vi "TagDB-Load.vi"(8 "error in (no error)":errorcluster, 9 "ignore internal data(T)":bool=TRUE, 10 "file path(empty for default)":path, 11 "DB Ref":refnum<k1>) -> (0 "error out":errorcluster, 1 "version":string, 3 "DB Ref(dup)":refnum<k1>)   [LabVIEW 2017, in "TagDB.lvlib"]
doc: "[Covers: REQ_API_Load]"
uses:
  TagDB.lvlib
  _Support/Disk/tagdbfile-v3.1.ctl
  _Support/Error/_Build Error Cluster.vi
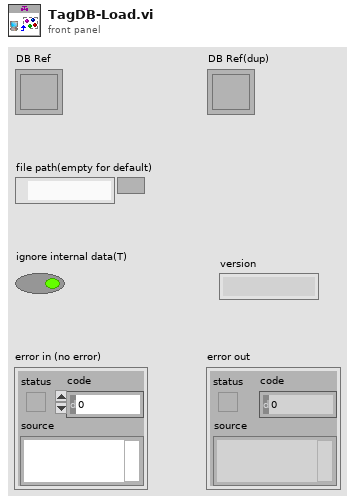
[diagram p1: front panel]
types:
  T1 = typedef "TagDB.lvlib/tagdbfile-v3.1.ctl" = cluster{"version":string, "db":variant[]}
  T2 = enum16{"open", "replace", "create", "open or create", "replace or create", "replace or create with confirmation"}
  T3 = typedef "TagDB.lvlib/tagdb-data.ctl" = cluster{"tag-map":variant, "timestamp-map":variant, "namecacher-map":variant, "DataTypeCacher-map":variant, "Tag Adding Lock?":bool, "Global Change Timestamp":timestamp, "Item Change Timestamp":timestamp, "name":string, "Global Change Flag":u64, "Item Change Flag":u64}
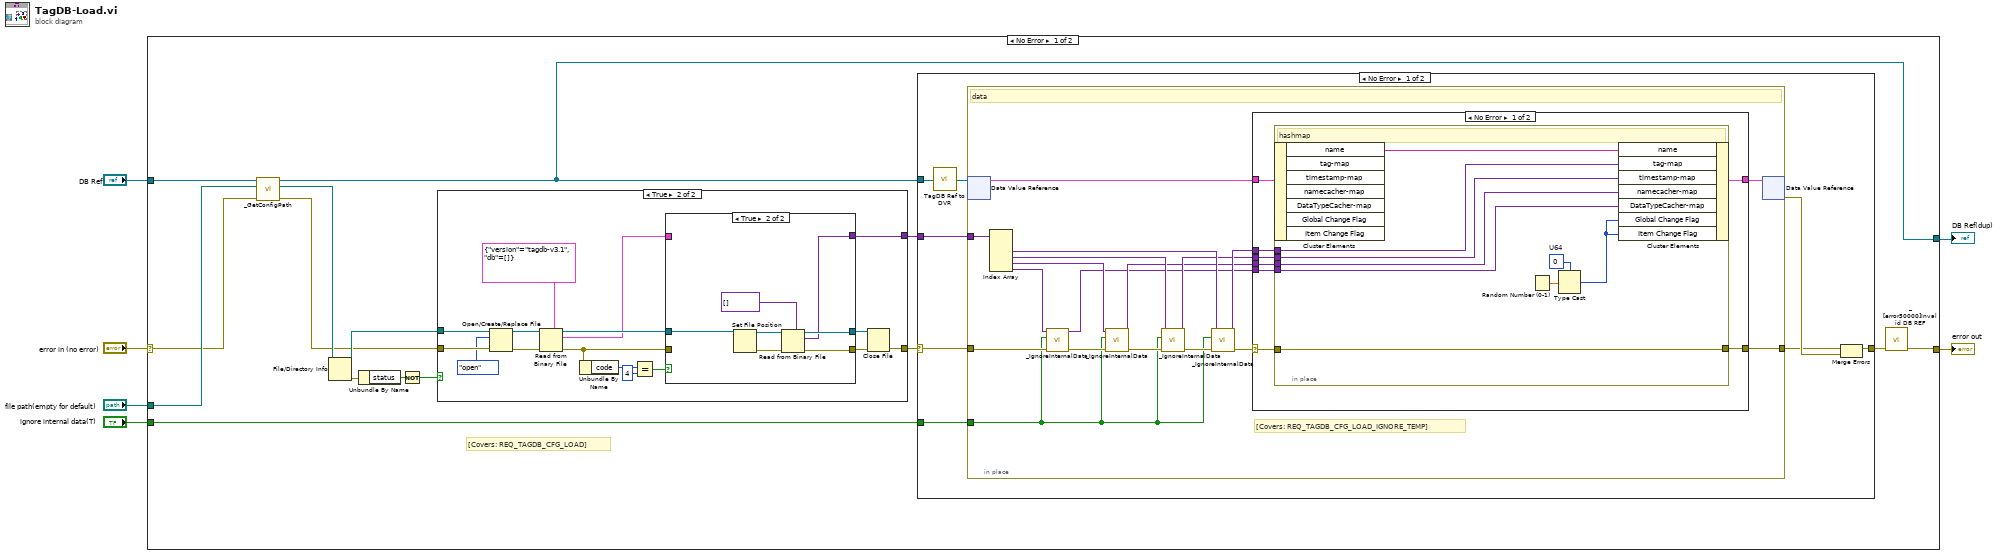
[diagram p0: block diagram]
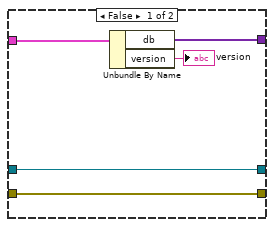
[diagram p5: hidden frame]
diagram:
  n1 = case shown="No Error" "error in (no error)" {
    selector: "error in (no error)" -> [w13 w98]
    tunnel: [w21 w98] -> w5
    tunnel: [w15 w97] -> w3
    tunnel: "DB Ref" -> [w14 w97]
    tunnel: "file path(empty for default)" -> [w16 _]
    tunnel: "ignore internal data(T)" -> [w20 _]
    frame No Error {
      # "[Covers: REQ_TAGDB_CFG_LOAD]"
      n2 = call "_GetConfigPath.vi"("error in (no error)"=w13, "file path(empty for default) in"=w16, "DB Ref"=w14) -> ("error out"=w8:errorcluster, "file path(empty for default) out"=w10:path, "DB Ref(dup)"=w15:refnum<k1>)  [unwired: 6 in]
      n3 = File/Directory Info(path=w10) -> (path out=w9:path, error out=w12:errorcluster)  [unwired: 1 in, 5 out]
      n4 = Unbundle By Name(w12) -> ("status"=w11:bool)
      n5 = Not(x=w11) -> (.not. x?=w7:bool)
      n6 = case shown="True" w7 {
        tunnel: w8 -> [w68 w84]
        tunnel: w9 -> [_ w83]
        tunnel: [_ w75] -> w19
        tunnel: [w68 w79] -> w17
        frame False {
        }
        frame True {
          n7 = Open/Create/Replace File(file path (use dialog)=w83, error in=w84, operation (0:open)=T2."open") -> (refnum out=w82:refnum<file>, error out=w81:errorcluster)  [unwired: 3 in, 1 out]
          n8 = Read from Binary File(5:T1 {"version"="tagdb-v3.1", "db"=[]} ("tagdb-file-v3.1"), 8:w81, 11:w82) -> (0:w72:errorcluster, 2:w74:T1, 3:w77:refnum<file>)  [unwired: 3 in, 1 out]
          n9 = Unbundle By Name(w72) -> ("code"=w71:i32)
          n10 = Equal?(x=w71, y=4) -> (x = y?=w69:bool)
          n11 = case shown="True" w69 {
            tunnel: [w89 w92] -> w78
            tunnel: w77 -> [w89 w96]
            tunnel: [w88 w93] -> w76
            tunnel: [w87 w90] -> w75
            tunnel: w74 -> [w86 _]
            tunnel: w72 -> [w88 _]
            frame False {
              n12 = Unbundle By Name(w86) -> ("db"=w87:variant[], "version"=→"version":string)
            }
            frame True {
              n13 = Set File Position(refnum=w96) -> (refnum out=w94:refnum<file>, error out=w95:errorcluster)  [unwired: 3 in]
              n14 = Read from Binary File(5:variant[] [] ("Array"), 8:w95, 11:w94) -> (0:w93:errorcluster, 2:w90:variant[], 3:w92:refnum<file>)  [unwired: 3 in, 1 out]
            }
          }
          n15 = Close File(refnum=w78, error in=w76) -> (error out=w79:errorcluster)  [unwired: 1 out]
        }
      }
      n16 = case shown="No Error" w17 {
        selector: w17 -> [w24 w67]
        tunnel: w20 -> [w29 _]
        tunnel: w19 -> [w27 _]
        tunnel: [w26 w67] -> w18
        tunnel: w15 -> [w22 _]
        frame No Error {
          n17 = call "TagDB Ref to DVR.vi"("TagDB"=w22) -> ("DVR"=w28:refnum<data-value>)  [unwired: 4 in]
          n18 = in-place "In Place Element Structure" {
            in-place-border: w27 -> [w45]
            in-place-border: w29 -> [w33]
            in-place-border: w24 -> [w40]
            in-place-border: [w42] -> w23
            # "[Covers: REQ_TAGDB_CFG_LOAD_IGNORE_TEMP]"
            # "data"
            n19 = in-place-dvr #1 ("Data Value Reference Read / Write Element")(w28) -> (w47:T3)  [unwired: 1 out]
            n20 = Index Array(array=w45) -> (element #2=w41:variant, element #3=w36:variant, element #4=w35:variant, element #5=w34:variant)  [unwired: 5 in, 1 out]
            n21 = call "_IgnoreInternalData.vi"("error in (no error)"=w40, "ignore internal data(T)"=w33, "Variant in"=w34) -> ("error out"=w39:errorcluster, "Variant out"=w30:variant)  [unwired: 7 in]
            n22 = call "_IgnoreInternalData.vi"("error in (no error)"=w39, "ignore internal data(T)"=w33, "Variant in"=w35) -> ("error out"=w38:errorcluster, "Variant out"=w31:variant)  [unwired: 7 in]
            n23 = call "_IgnoreInternalData.vi"("error in (no error)"=w38, "ignore internal data(T)"=w33, "Variant in"=w36) -> ("error out"=w37:errorcluster, "Variant out"=w32:variant)  [unwired: 7 in]
            n24 = call "_IgnoreInternalData.vi"("error in (no error)"=w37, "ignore internal data(T)"=w33, "Variant in"=w41) -> ("error out"=w43:errorcluster, "Variant out"=w44:variant)  [unwired: 7 in]
            n25 = case shown="No Error" w43 {
              selector: w43 -> [w52 w65]
              tunnel: w47 -> [w55 w66]
              tunnel: [w54 w66] -> w46
              tunnel: w44 -> [w53 _]
              tunnel: [w51 w65] -> w42
              tunnel: w32 -> [w50 _]
              tunnel: w31 -> [w49 _]
              tunnel: w30 -> [w48 _]
              frame No Error {
                n26 = in-place "In Place Element Structure" {
                  in-place-border: w53 -> [w63]
                  in-place-border: w52 -> [w64]
                  in-place-border: [w64] -> w51
                  in-place-border: w50 -> [w62]
                  in-place-border: w49 -> [w61]
                  in-place-border: w48 -> [w60]
                  w57 = u64 0  # U64
                  # "hashmap"
                  n27 = in-place-cluster #2 ("Unbundle / Bundle Elements")(w55) -> ("name"=w59:string)  [unwired: 6 out]
                  n28 = Random Number (0-1)() -> (number: 0 to 1=w58:dbl)
                  n29 = Type Cast(type=w57, x=w58) -> (*(type *) &x=w56:u64)
                  n30 = in-place-cluster #2 ("Unbundle / Bundle Elements")("name"=w59, "tag-map"=w63, "timestamp-map"=w62, "namecacher-map"=w61, "DataTypeCacher-map"=w60, "Global Change Flag"=w56, "Item Change Flag"=w56) -> (w54:T3)
                }
              }
              frame Error {
              }
            }
            n31 = in-place-dvr #1 ("Data Value Reference Read / Write Element")(w46) -> (w25:errorcluster)  [unwired: 1 out]
          }
          n32 = Merge Errors(w23, w25) -> (w26:errorcluster)
        }
        frame Error {
        }
      }
      n33 = call "_[error50000]Invalid DB REF.vi"("error in (no error)"=w18) -> ("error out"=w21:errorcluster)  [unwired: 10 in]
    }
    frame Error {
    }
  }
  "error out" <- w5
  "DB Ref(dup)" <- w3
